vi "Persist New Entity.vi"(8 "error in (no error)":errorcluster, 9 "Entity":refnum<class "Entity.lvclass">, 10 "Types":refnum<class "Type.lvclass">[](array[class]), 11 "Database in":refnum<class "Database Platform.lvclass">) -> (0 "error out":errorcluster, 2 "New ID":T1, 3 "Database out":refnum<class "Database Platform.lvclass">)   [LabVIEW 2020, in "Conditu2.lvlib" / "Database Platform.lvclass"]
uses:
  Database Platform.lvclass
  Entity/Entity.lvclass
  Entity ID.ctl
  Columns/Type/Type.lvclass
  Conditu2.lvlib
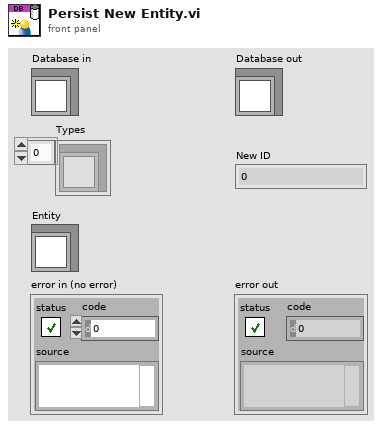
[diagram p1: front panel]
types:
  T1 = typedef "Conditu2.lvlib/Entity ID.ctl" = i64
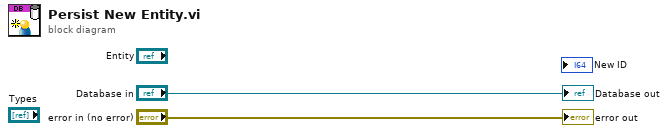
[diagram p0: block diagram]
diagram:
  "error out" <- "error in (no error)"
  "Database out" <- "Database in"
